vi "APC_PC_SlaveModbus.vi"() -> ()   [LabVIEW 2020]
doc: "Demonstrates how to use Modbus functions to create a slave listening to a specific TCP port. It shows an interactive UI to allow users read and write the coils on a virtual slave device. Users can also get the count of masters connected to this slave."
uses:
  <vilib>/Modbus/slave/Create Slave Instance (TCP).vi
  <vilib>/Modbus/slave/Modbus Slave.lvclass
panel:
  in  "holding register values":u16[](array[numeric])
  out "Number of Masters":u32
  in  "Get TCP Connection Count":bool
  in  "Read Count":u16=10
  in  "Stop":bool
  in  "Read":bool
  out "Coil Values Read":bool[](array[boolean])
  in  "Write":bool
  in  "Coil Values to Write":bool[](array[boolean])
  # "Overview: Demonstrates the use of the Modbus Slave VIs to create a Modbus slave and read and write coil values on this Modbus slave.\nRequirements: LabVIEW Datalogging and Supervisory Control Module\nInstructions:\n1. Ensure Port 502 is not in use.\n2. Run the VI.\n3. Click Stop to stop the VI."
  # "Write Operation"
  # "Read Operation"
  # "Get Number Of Masters"
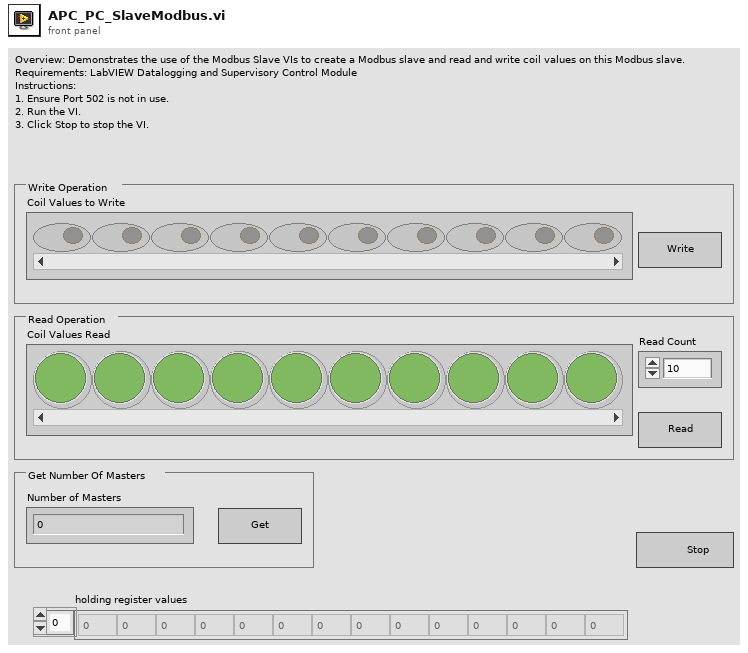
[diagram p1: front panel]
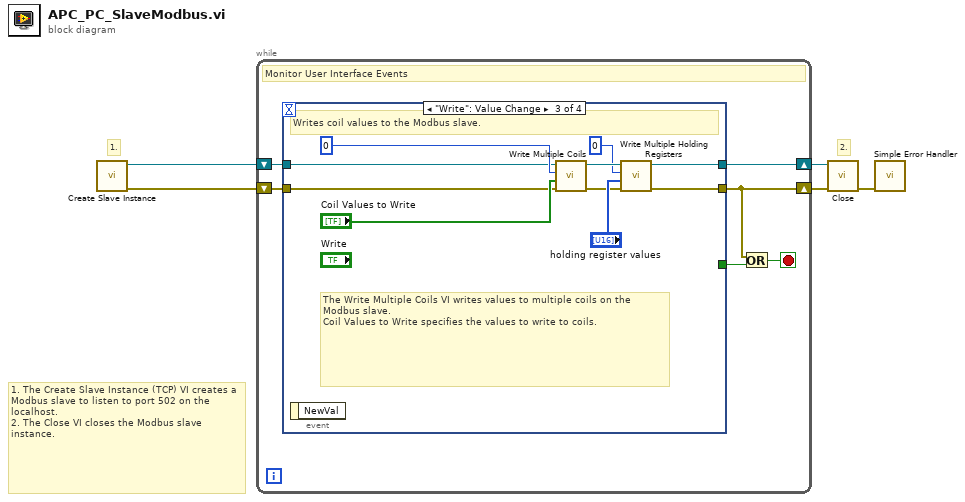
[diagram p0: block diagram]
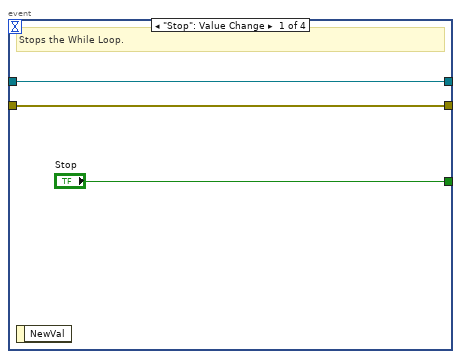
[diagram p2: hidden frame]
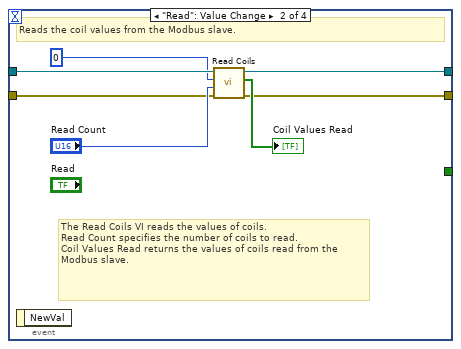
[diagram p3: hidden frame]
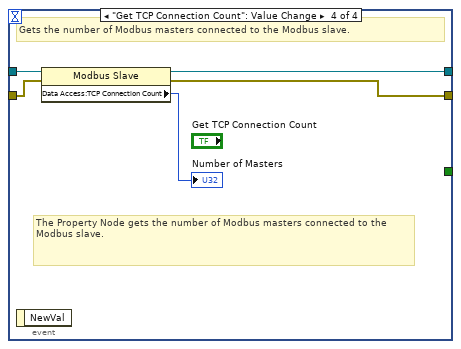
[diagram p4: hidden frame]
diagram:
  # "2."
  # "1."
  # "1. The Create Slave Instance (TCP) VI creates a Modbus slave to listen to port 502 on the localhost.\n2. The Close VI closes the Modbus slave instance."
  n1 = call-poly <vilib>:"Create Slave Instance.vi"() -> ("error out"=w4:errorcluster, "TCP slave instance"=w5:refnum<class "Modbus Slave.lvclass">)  [unwired: 10 in]
  n2 = while {
    shift-right: [w10] -> w2
    shift-left: w5 -> [w11]
    shift-right: [w8] -> w3
    shift-left: w4 -> [w9]
    stop <- w6 stop-if-true
    # "Monitor User Interface Events"
    n3 = event shown="[2] \"Write\": Value Change" {
      selector: _ -> [_ _ _ _]
      dyn-events: _ -> [_ _ _ _]
      timeout: _ -> [_ _ _ _]
      tunnel: ["Stop" _ _ _] -> w7
      tunnel: w11 -> [w13 w21 w29 w36]
      tunnel: [w13 w20 w23 w34] -> w10
      tunnel: w9 -> [w14 w16 w28 w35]
      tunnel: [w14 w15 w22 w32] -> w8
      event "Stop": Value Change {
        # "Stops the While Loop."
        n4 = event-data() -> ()  [unwired: 1 in, 1 out]
      }
      event "Read": Value Change {
        # "The Read Coils VI reads the values of coils.\nRead Count specifies the number of coils to read.\nCoil Values Read returns the values of coils read from the Modbus slave."
        # "Reads the coil values from the Modbus slave."
        n5 = event-data() -> ()  [unwired: 1 in, 1 out]
        n6 = call-dynamic "Read Coils.vi"("error in (no error)"=w16, "number of coils"="Read Count", "starting address"=u16 0, "Modbus slave in"=w21) -> ("error out"=w15:errorcluster, "coil values"=→"Coil Values Read":bool[], "Modbus slave out"=w20:refnum<class "Modbus Slave.lvclass">)  [unwired: 5 in]
      }
      event "Write": Value Change {
        # "The Write Multiple Coils VI writes values to multiple coils on the Modbus slave.\nCoil Values to Write specifies the values to write to coils."
        # "Writes coil values to the Modbus slave."
        n7 = event-data() -> ()  [unwired: 1 in, 1 out]
        n8 = call-dynamic "Write Multiple Coils.vi"("error in (no error)"=w28, "coil values"="Coil Values to Write", "starting address"=u16 0, "Modbus slave in"=w29) -> ("error out"=w24:errorcluster, "Modbus slave out"=w27:refnum<class "Modbus Slave.lvclass">)  [unwired: 6 in]
        n9 = call-dynamic "Write Multiple Holding Registers.vi"("error in (no error)"=w24, "holding register values"="holding register values", "starting address"=u16 0, "Modbus slave in"=w27) -> ("error out"=w22:errorcluster, "Modbus slave out"=w23:refnum<class "Modbus Slave.lvclass">)  [unwired: 6 in]
      }
      event "Get TCP Connection Count": Value Change {
        # "The Property Node gets the number of Modbus masters connected to the Modbus slave."
        # "Gets the number of Modbus masters connected to the Modbus slave."
        n10 = event-data() -> ()  [unwired: 1 in, 1 out]
        n11 = property class="Modbus Slave"(reference=w36, error in=w35) -> (reference out=w34:refnum<class "Modbus Slave.lvclass">, error out=w32:errorcluster, "Data Access:TCP Connection Count"=→"Number of Masters":u32)
      }
    }
    n12 = Or(x=w8, y=w7) -> (x .or. y?=w6:bool)
  }
  n13 = call-dynamic "Close.vi"("error in (no error)"=w3, "Modbus slave in"=w2) -> ("error out"=w1:errorcluster)  [unwired: 9 in]
  n14 = call <vilib>:"Simple Error Handler.vi"("error in (no error)"=w1) -> ()  [unwired: 4 in, 5 out]
